vi "GetPositionAll.vi"(8 "PicError":errorcluster, 9 "StepError":errorcluster, 10 "CmdLib In":refnum<k24>, 11 "com in":refnum<visa-resource-name>) -> (0 "PicErrorOut":errorcluster, 1 "StepError":errorcluster caption="StepErrorOut", 2 "CmdLib Out":refnum<k24>, 3 "com out":refnum<visa-resource-name>, 4 "PositionOut":i32[](array[numeric]))   [LabVIEW 2018]
uses:
  Device VIs/CmdLib.dll
  Device VIs/Verbal.vi
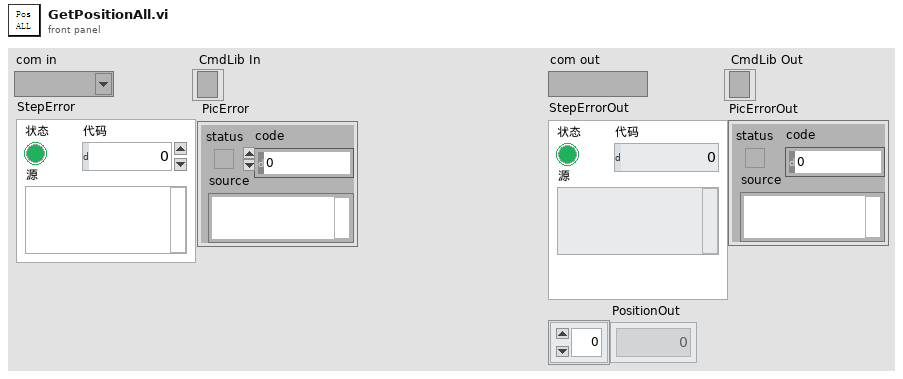
[diagram p1: front panel]
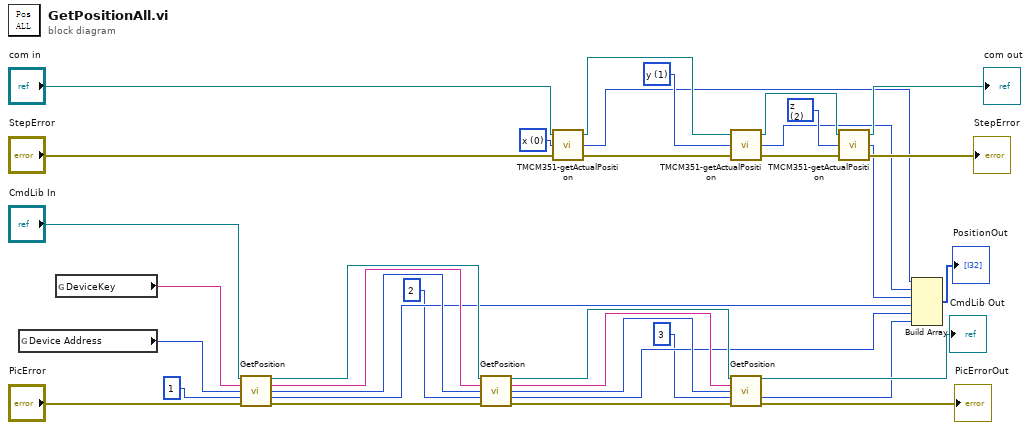
[diagram p0: block diagram]
diagram:
  w19 = u8 2 items=["x", "y", "z"] ("motor")
  w20 = u8 1 items=["x", "y", "z"] ("motor")
  w21 = u8 0 items=["x", "y", "z"] ("motor")
  n1 = global read "Verbal.vi" "Device Address"() -> (w1:i32)
  n2 = global read "Verbal.vi" "DeviceKey"() -> (w2:string)
  n3 = call "GetPosition.vi"("CmdLib In"="CmdLib In", "DeviceKey In"=w2, "Device Address In"=w1, "Motor"=1, "error in (no error)"="PicError") -> ("CmdLib Out"=w29:refnum<k24>, "DeviceKey Out"=w27:string, "Device Address Out"=w26:i32, "Position"=w9:i32, "error out"=w28:errorcluster)  [unwired: 6 in]
  n4 = call "GetPosition.vi"("CmdLib In"=w29, "DeviceKey In"=w27, "Device Address In"=w26, "Motor"=2, "error in (no error)"=w28) -> ("CmdLib Out"=w25:refnum<k24>, "DeviceKey Out"=w24:string, "Device Address Out"=w23:i32, "Position"=w8:i32, "error out"=w22:errorcluster)  [unwired: 6 in]
  n5 = call "TMCM351-getActualPosition.vi"("错误输入"="StepError", "motor"=w21, "com in"="com in") -> ("错误输出"=w33:errorcluster, "Pisotion"=w12:i32, "com out"=w32:refnum<visa-resource-name>)
  n6 = call "TMCM351-getActualPosition.vi"("错误输入"=w33, "motor"=w20, "com in"=w32) -> ("错误输出"=w31:errorcluster, "Pisotion"=w11:i32, "com out"=w30:refnum<visa-resource-name>)
  n7 = call "GetPosition.vi"("CmdLib In"=w25, "DeviceKey In"=w24, "Device Address In"=w23, "Motor"=3, "error in (no error)"=w22) -> ("CmdLib Out"=→"CmdLib Out":refnum<k24>, "Position"=w7:i32, "error out"=→"PicErrorOut":errorcluster)  [unwired: 6 in, 2 out]
  n8 = call "TMCM351-getActualPosition.vi"("错误输入"=w31, "motor"=w19, "com in"=w30) -> ("错误输出"=→"StepError":errorcluster, "Pisotion"=w10:i32, "com out"=→"com out":refnum<visa-resource-name>)
  n9 = Build Array(w12, w11, w10, w9, w8, w7) -> (→"PositionOut":i32[])
